vi "Send Press Transaction.vi"(7 "Message Priority (Normal)":T2=enum."Normal", 8 "error in (no error)":errorcluster, 10 "Transactions":T1, 11 "Message Enqueuer":refnum<class "Message Enqueuer.lvclass">) -> (0 "error out":errorcluster, 3 "Message Enqueuer out":refnum<class "Message Enqueuer.lvclass">)   [LabVIEW 2019, in "ATM Controller.lvlib" / "Press Transaction Msg.lvclass"]
doc: "This VI sends the message to an actor."
uses:
  Press Transaction Msg.lvclass
  <vilib>/ActorFramework/Message Enqueuer/Message Enqueuer.lvclass
  <vilib>/ActorFramework/Message Enqueuer/Message Priority.ctl
  Simulated User Console Actor/Simulated User Console Actor/Transactions -Cluster.ctl
  C:/Program Files (x86)/National Instruments/LabVIEW 2019/vi.lib/ActorFramework/Message/Message.lvclass
  Press Transaction Msg.lvclass/Press Transaction Msg.ctl
  <vilib>/ActorFramework/Message Enqueuer/Message Enqueuer.lvclass/Message Enqueuer.ctl
  <vilib>/ActorFramework/Message Priority Queue/Priority Enqueue.vi
  Simulated User Console Actor/Simulated User Console Actor/Simulated User Console Actor.lvclass
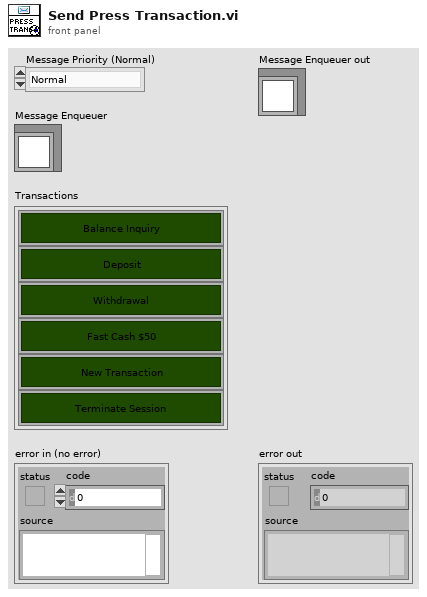
[diagram p1: front panel]
types:
  T1 = typedef "Simulated User Console Actor.lvlib/Simulated User Console Actor.lvclass/Transactions -Cluster.ctl" = cluster{"Balance Inquiry":bool, "Deposit":bool, "Withdrawal":bool, "Fast Cash $50":bool, "New Transaction":bool, "Terminate Session":bool}
  T2 = typedef "Actor Framework.lvlib/Message Enqueuer.lvclass/Message Priority.ctl" = enum16{"Low", "Normal", "High"}
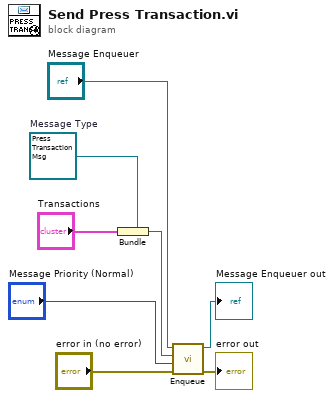
[diagram p0: block diagram]
diagram:
  w2 = refnum<class "Press Transaction Msg.lvclass"> refnum  # Message Type
  n1 = Bundle(cluster=w2, "Transactions") -> (w3:refnum<class "Press Transaction Msg.lvclass">)
  n2 = call <vilib>:"Enqueue.vi"("error in (no error)"="error in (no error)", "Message Priority (Normal)"="Message Priority (Normal)", "Message"=w3, "Message Enqueuer in"="Message Enqueuer") -> ("error out"=→"error out":errorcluster, "Message Enqueuer out"=→"Message Enqueuer out":refnum<class "Message Enqueuer.lvclass">)  [unwired: 6 in]
